vi "23384_Davis_Poku_Amankwa_Amankwa.DavisPoku.MNE1201.3.DIY_348255_1831073681.vi"() -> ()   [LabVIEW 2018]
uses:
  <vilib>/Analysis/NI_AALBase.lvlib
panel:
  out "Waveform Graph":i32[](graph)
  in  "Total number of Trials":dbl
  out "Number of Heads":dbl
  out "Coin 4":bool
  out "Coin 3":bool
  out "Coin 2":bool
  out "Coin 1":bool
  # "Consistency with the Stastistical expectation is Observed when N is  approximately greater than 100"
  # "Heads =Lit"
  # "Tails = Unlit"
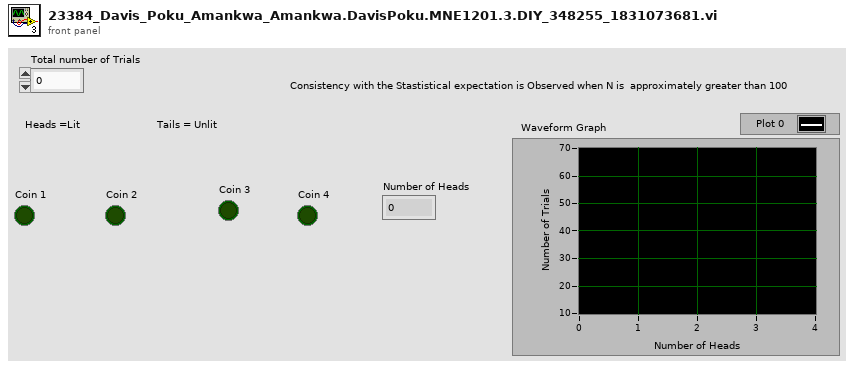
[diagram p1: front panel]
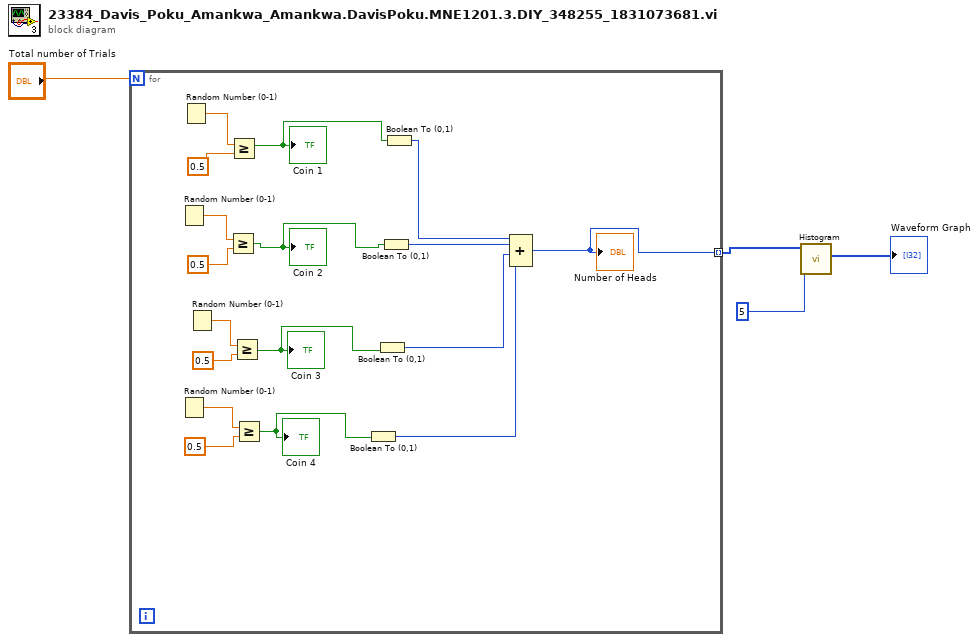
[diagram p0: block diagram]
diagram:
  n1 = for {
    N: "Total number of Trials" -> [_]
    tunnel: [w6] -> w2 mode=indexing
    n2 = Random Number (0-1)() -> (number: 0 to 1=w20:dbl)
    n3 = Random Number (0-1)() -> (number: 0 to 1=w16:dbl)
    n4 = Random Number (0-1)() -> (number: 0 to 1=w5:dbl)
    n5 = Random Number (0-1)() -> (number: 0 to 1=w18:dbl)
    n6 = Greater Or Equal?(x=w20, y=0.5) -> (x >= y?=w11:bool)
    "Coin 2" <- w11
    n7 = Greater Or Equal?(x=w5, y=0.5) -> (x >= y?=w12:bool)
    "Coin 1" <- w12
    n8 = Greater Or Equal?(x=w18, y=0.5) -> (x >= y?=w14:bool)
    "Coin 3" <- w14
    n9 = Greater Or Equal?(x=w16, y=0.5) -> (x >= y?=w13:bool)
    "Coin 4" <- w13
    n10 = Boolean To (0,1)(Boolean=w13) -> (0, 1=w9:i16)
    n11 = Boolean To (0,1)(Boolean=w14) -> (0, 1=w10:i16)
    n12 = Boolean To (0,1)(Boolean=w11) -> (0, 1=w8:i16)
    n13 = Boolean To (0,1)(Boolean=w12) -> (0, 1=w7:i16)
    n14 = Compound Arithmetic op=ADD(w7, w8, w10, w9) -> (w6:i16)
    "Number of Heads" <- w6
  }
  n15 = call <vilib>:"Histogram.vi"("intervals"=5, "X"=w2) -> ("Histogram: h(x)"=→"Waveform Graph":i32[])  [unwired: 6 in, 3 out]
